vi "Update Trace Tree.vi"(7 "References":T1, 8 "error in":errorcluster, 10 "Headers":string[](array[string]), 11 "Data IN":string[][](array[string])) -> (0 "error out":errorcluster, 2 "Signals":string[][](table))   [LabVIEW 2025, in "CAN-LIN Raw Bus Capture UI.lvlib"]
doc: "This VI processes the DATA and populates the Frame TREE and the Signal TABLE."
uses:
  CAN-LIN Raw Bus Capture UI.lvlib
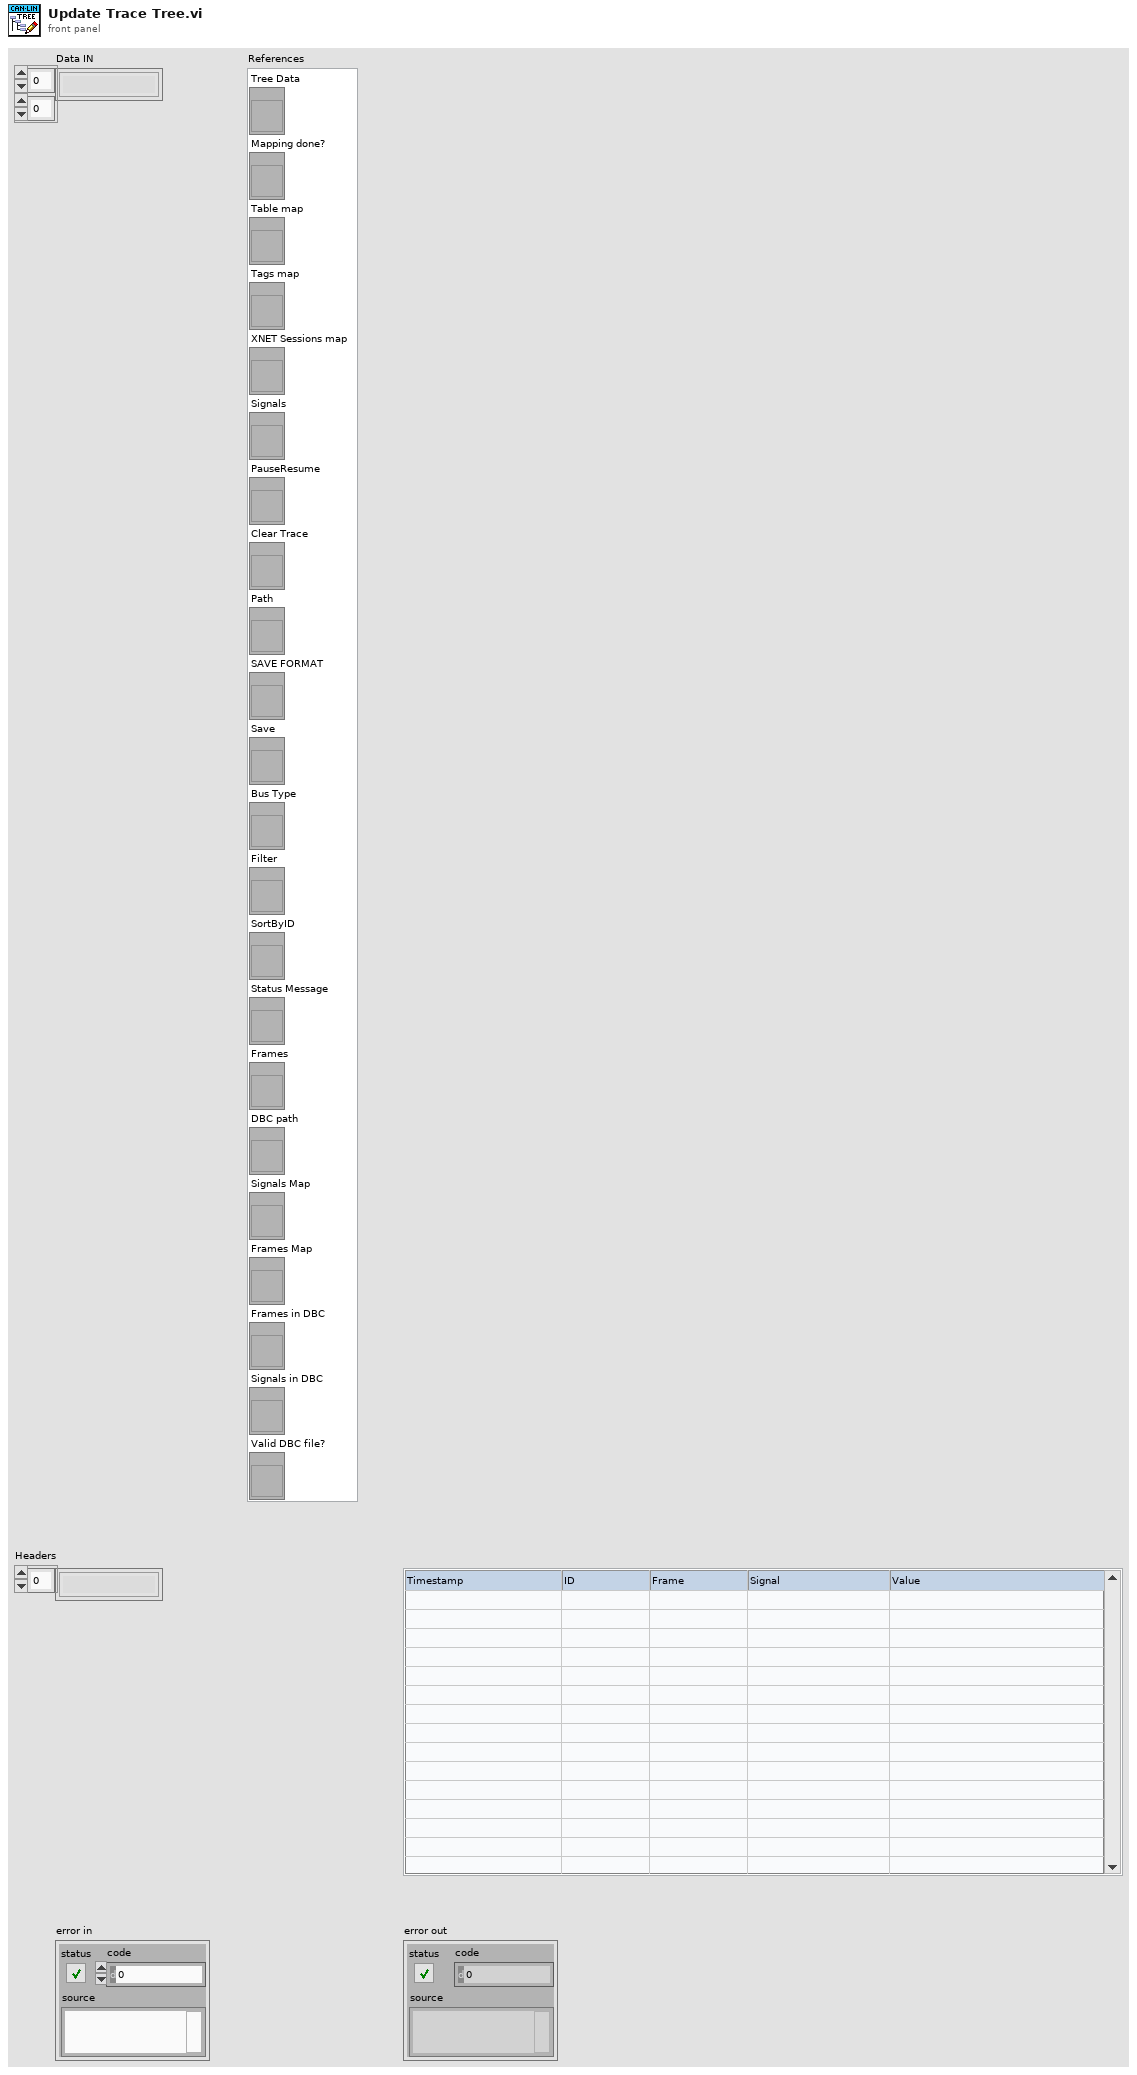
[diagram p1: front panel]
types:
  T1 = cluster{"Tree Data":refnum<vi>, "Mapping done?":refnum<vi>, "Table map":refnum<vi>, "Tags map":refnum<vi>, "XNET Sessions map":refnum<vi>, "Signals":refnum<vi>, "PauseResume":refnum<vi>, "Clear Trace":refnum<vi>, "Path":refnum<vi>, "SAVE FORMAT":refnum<vi>, "Save":refnum<vi>, "Bus Type":refnum<vi>, "Filter":refnum<vi>, "SortByID":refnum<vi>, "Status Message":refnum<vi>, "Frames":refnum<vi>, "DBC path":refnum<vi>, "Signals Map":refnum<vi>, "Frames Map":refnum<vi>, "Frames in DBC":refnum<vi>, "Signals in DBC":refnum<vi>, "Valid DBC file?":refnum<vi>}
  T2 = typedef "XNET Frame CAN.ctl" = cluster{"timestamp":timestamp, "payload":u8[], "identifier":u32, "type":T3, "extended?":bool, "echo?":bool}
  T3 = typedef "XNET Frame Type CAN.ctl" = u8
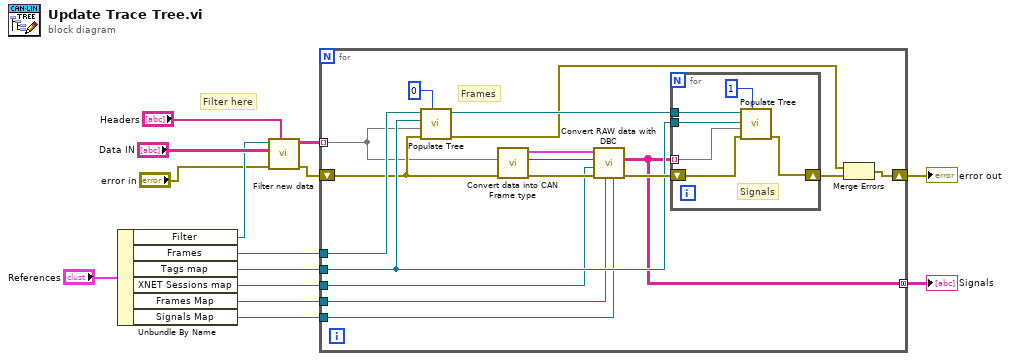
[diagram p0: block diagram]
diagram:
  # "Filter here"
  n1 = Unbundle By Name("References") -> ("Filter"=w3:refnum<vi>, "Frames"=w12:refnum<vi>, "Tags map"=w8:refnum<vi>, "XNET Sessions map"=w10:refnum<vi>, "Frames Map"=w9:refnum<vi>, "Signals Map"=w11:refnum<vi>)
  n2 = call "Filter new data.vi"("Headers"="Headers", "error in"="error in", "Data IN"="Data IN", "String in"=w3) -> ("error out"=w4:errorcluster, "Filtered Array"=w5:string[][])  [unwired: 6 in]
  n3 = for {
    tunnel: w5 -> [w15] mode=indexing
    tunnel: w12 -> [w23]
    tunnel: [w26] -> w14 mode=concatenating
    shift-right: [w28] -> w13
    shift-left: w4 -> [w20]
    tunnel: w9 -> [w25]
    tunnel: w11 -> [w24]
    tunnel: w8 -> [w27]
    tunnel: w10 -> [w17]
    # "Frames"
    n4 = call "Populate Tree.vi"("Indent level"=0 ("Numeric"), "error in"=w20, "Data in"=w15, "Tags map"=w27, "TreeControl in"=w23) -> ("error out"=w22:errorcluster)  [unwired: 6 in]
    n5 = call "Convert data into CAN Frame type.vi"("error in"=w20, "Frame"=w15) -> ("error out"=w19:errorcluster, "ID"=w30:u32, "CAN frame"=w18:T2)  [unwired: 7 in]
    n6 = call "Convert RAW data with DBC.vi"("Signals Map"=w24, "Frames Map"=w25, "error in"=w19, "XNET Sessions map"=w17, "ID"=w30, "Frame"=w18) -> ("error out"=w29:errorcluster, "Human Readable DATA"=w26:string[][])  [unwired: 4 in]
    n7 = for {
      tunnel: w26 -> [w31] mode=indexing
      tunnel: w23 -> [w36]
      shift-right: [w34] -> w21
      shift-left: w29 -> [w35]
      tunnel: w27 -> [w33]
      # "Signals"
      n8 = call "Populate Tree.vi"("Indent level"=1, "error in"=w35, "Data in"=w31, "Tags map"=w33, "TreeControl in"=w36) -> ("error out"=w34:errorcluster)  [unwired: 6 in]
    }
    n9 = Merge Errors(w22, w21) -> (w28:errorcluster)
  }
  "Signals" <- w14
  "error out" <- w13
